vi "Greet World.vi"(7 "Hello (T)/Goodbye(F)":bool, 8 "error in (no error)":errorcluster, 11 "English in":refnum<class "English.lvclass">) -> (0 "error out":errorcluster, 2 "Greeting String":string, 3 "English out":refnum<class "English.lvclass">)   [LabVIEW 2019, in "English.lvclass"]
uses:
  English.lvclass
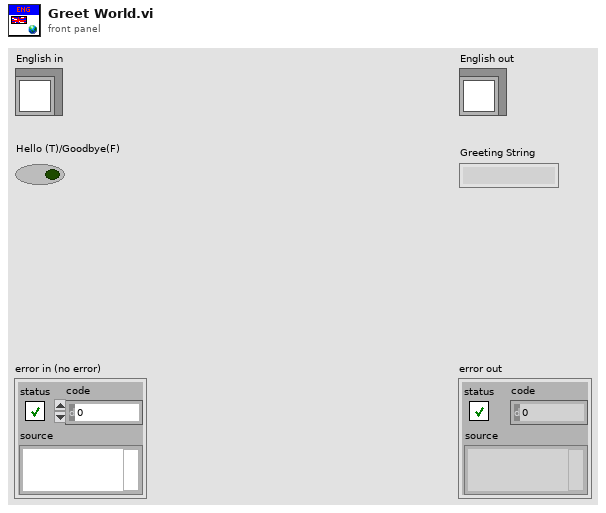
[diagram p1: front panel]
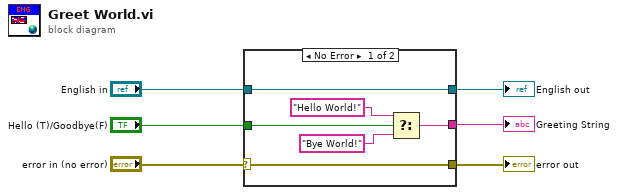
[diagram p0: block diagram]
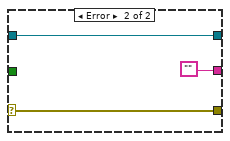
[diagram p2: hidden frame]
diagram:
  n1 = case shown="No Error" "error in (no error)" {
    selector: "error in (no error)" -> [w12 w15]
    tunnel: [w12 w15] -> w5
    tunnel: [w11 w14] -> w4
    tunnel: "English in" -> [w11 w14]
    tunnel: "Hello (T)/Goodbye(F)" -> [w10 _]
    tunnel: [w9 ""] -> w1
    frame No Error {
      n2 = Select(t="Hello World!", s=w10, f="Bye World!") -> (s? t:f=w9:string)
    }
    frame Error {
    }
  }
  "error out" <- w5
  "English out" <- w4
  "Greeting String" <- w1
